vi "Route Throttle AIs.vi"(0 "ThrottleDataToControl":T1, 5 "ExternalAI1":sgl, 7 "ExternalAI2":sgl, 9 "UseExtAI1":bool, 11 "UseExtAI2":bool) -> (8 "ThrottleDataToControl":T1)   [LabVIEW 2015, in "ECS-RT.lvlib"]
uses:
  ECS-RT.lvlib
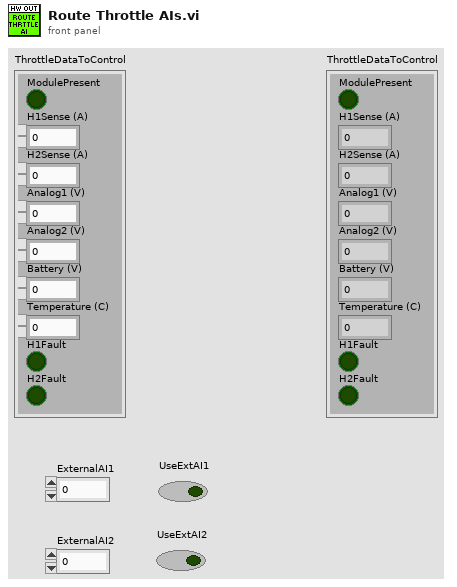
[diagram p1: front panel]
types:
  T1 = cluster{"ModulePresent":bool, "H1Sense (A)":sgl, "H2Sense (A)":sgl, "Analog1 (V)":sgl, "Analog2 (V)":sgl, "Battery (V)":sgl, "Temperature (C)":sgl, "H1Fault":bool, "H2Fault":bool}
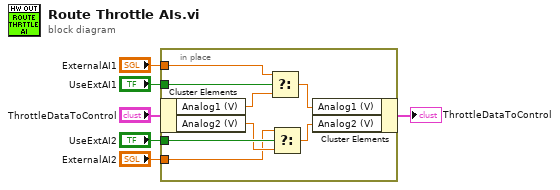
[diagram p0: block diagram]
diagram:
  n1 = in-place {
    in-place-border: "UseExtAI1" -> [w13]
    in-place-border: "UseExtAI2" -> [w14]
    in-place-border: "ExternalAI1" -> [w12]
    in-place-border: "ExternalAI2" -> [w8]
    n2 = in-place-cluster #1("ThrottleDataToControl") -> ("Analog1 (V)"=w11:sgl, "Analog2 (V)"=w9:sgl)
    n3 = Select(t=w12, s=w13, f=w11) -> (s? t:f=w10:sgl)
    n4 = Select(t=w8, s=w14, f=w9) -> (s? t:f=w7:sgl)
    n5 = in-place-cluster #1("Analog1 (V)"=w10, "Analog2 (V)"=w7) -> (→"ThrottleDataToControl":T1)
  }
